vi "drivable_paths_notimer.vi"(2 "y LIDAR position":i16, 3 "x LIDAR position":i16, 4 "number 16\" iterations":i32) -> (0 "max distance":i16[](array[numeric]))   [LabVIEW 2009]
uses:
  <vilib>/Platform/TimedLoop/XDataNode/XDataNode.xnode
  <vilib>/Platform/TimedLoop/XDataNode/loadlvalarms.vi
  <vilib>/Platform/TimedLoop/XDataNode/timing_clust.ctl
  <vilib>/Platform/TimedLoop/XDataNode/nitl_modes.ctl
  <vilib>/Platform/TimedLoop/XDataNode/wakeup.ctl
  <vilib>/Platform/TimedLoop/XDataNode/XDNodeRunTimeDep.lvlib
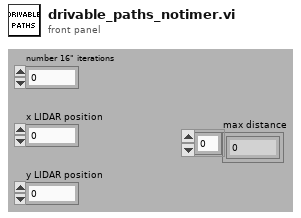
[diagram p1: front panel]
types:
  T1 = typedef "XDNodeRunTimeDep.lvlib/timing_clust.ctl" = cluster{"Expected End [f-1]":u64, "Actual End [f-1]":u64, "Finished Late? [f-1]":bool, "Expected End [i-1]":u64, "Actual End [i-1]":u64, "Finished Late? [i-1]":bool, "Expected Start [i]":u64, "Actual Start [i]":u64, "Expected Start [f]":u64, "Actual Start [f]":u64, "Source Name":string, "Structure Name":string, "Period":i64, "Deadline":i64, "Offset":i64, "Start":i64, "Priority":i32, "Timeout":i32, "Mode":T2, "Wakeup Reason":T3, "Error":errorcluster, "Source Type":string, "Secondary Source Type":string, "Global End Time":u64, "Global Start Time":u64, "Frame Duration":u64, "Iteration Duration":u64, "Assigned CPU":i32, "I/O Scan Engine Mode":u32}
  T2 = typedef "XDNodeRunTimeDep.lvlib/nitl_modes.ctl" = enum32{"No Change", "Process missed periods, maintain original phase", "Discard missed periods, maintain original phase", "Process missed periods, ignore original phase", "Discard missed periods, ignore original phase"}
  T3 = typedef "XDNodeRunTimeDep.lvlib/wakeup.ctl" = enum32{"Normal", "Aborted", "Asynchronous wakeup", "Timing source error", "Timed loop error", "Timeout"}
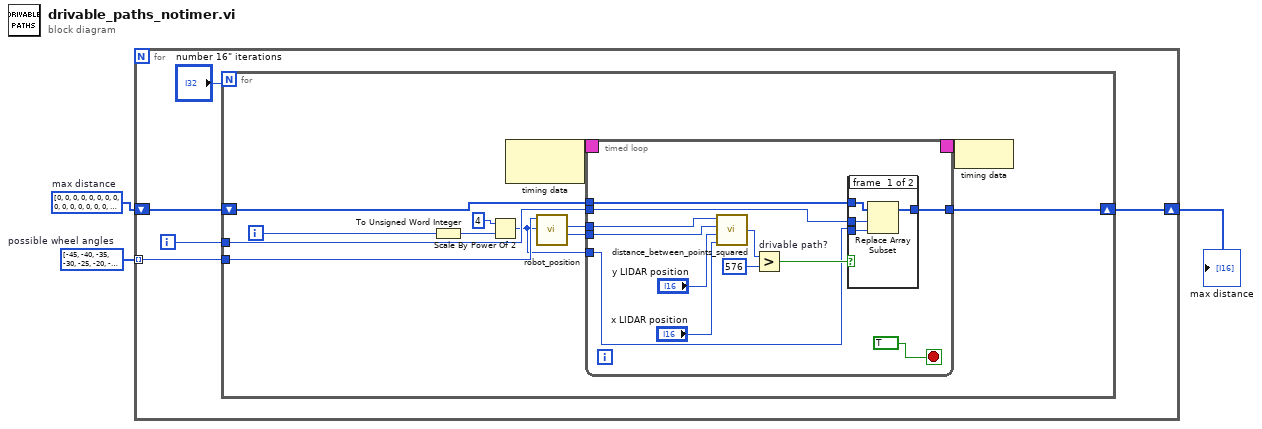
[diagram p0: block diagram]
diagram:
  w2 = i8[] [-45, -40, -35, -30, -25, -20, -15, -10, -5, 0, 5, 10, 15, 20, 25, 30, 35, 40, 45]  # possible wheel angles
  w1 = i16[] [0, 0, 0, 0, 0, 0, 0, 0, 0, 0, 0, 0, 0, 0, 0, 0, 0, 0, 0]  # max distance
  n1 = for {
    tunnel: w2 -> [w7] mode=indexing
    shift-right: [w5] -> w3
    shift-left: w1 -> [w8]
    i -> [w6]
    n2 = for {
      N: "number 16\" iterations" -> [_]
      tunnel: w6 -> [w17]
      tunnel: w7 -> [w16]
      shift-right: [w18] -> w5
      shift-left: w8 -> [w20]
      i -> [w19]
      n3 = To Unsigned Word Integer(number=w19) -> (unsigned 16bit integer=w14:u16)
      n4 = Scale By Power Of 2(n=u16 4, x=w14) -> (x*2^n=w9:u16)
      n5 = node-c288() -> (w11:T1)  [unwired: 1 in]
      n6 = call "robot_position.vi"("Distance Along Arc"=w9, "Wheel Angle"=w16) -> ("New X Position"=w13:i8, "New Y Position"=w12:i8)  [unwired: 7 in, 1 out]
      n7 = timed-loop {
        timing: w11 -> [_]
        timing-out: [_] -> w10
        tunnel: w20 -> [w32]
        tunnel: [w31] -> w18
        tunnel: w17 -> [w30]
        tunnel: w13 -> [w29]
        tunnel: w12 -> [w28]
        tunnel: w9 -> [w21]
        stop <- TRUE stop-if-true
        n8 = call "distance_between_points_squared.vi"("x LIDAR position"="x LIDAR position", "y LIDAR position"="y LIDAR position", "x position"=w29, "y position"=w28) -> ("distance squared"=w23:i16)  [unwired: 2 in]
        n9 = Greater? "drivable path?"(x=w23, y=i16 576) -> (0:w24:bool)
        n10 = case shown="False" w24 {
          tunnel: w32 -> [w36 w37]
          tunnel: w21 -> [w35 _]
          tunnel: [w34 w37] -> w31
          tunnel: w30 -> [w33 _]
          frame #0 {
            n11 = Replace Array Subset(array=w36, new element=w35, index=w33) -> (w34:i16[])
          }
          frame #1 {
          }
        }
      }
      n12 = node-c288(w10) -> ()
    }
  }
  "max distance" <- w3
